vi "ModeloSegundoOrden.vi"() -> ()   [LabVIEW 2019]
uses:
  <vilib>/addons/Control Design/_Model Construction/Special Model Creation.llb/Special Model Creation SubVI/CD Create 2nd Order Model.vi
  <vilib>/addons/Control Design/_Utility/Model Viewer.llb/Model Viewer SubVI/cd_Draw Zero-Pole-Gain Equation (TF).vi
  <vilib>/addons/Control Design/_Utility/Model Viewer.llb/Model Viewer SubVI/cd_Draw Transfer Function Equation (TF).vi
  <vilib>/addons/control/pid/pid.llb/PID (DBL).vi
  <vilib>/addons/control/pid/NI_PID_pid.lvlib
  <vilib>/addons/Control Design/_Model Construction/NI_CD_Special Model Creation.lvlib
  <vilib>/addons/Control Design/_Utility/NI_CD_Model Viewer.lvlib
panel:
  out "Equation 2":picture
  in  "Natural Frequency (rad/s)":dbl format="%.4f"
  in  "stop":bool
  in  "paso (s)":dbl
  in  "PID gains":T1={"proportional gain (Kc)"=1.0, "integral time (Ti, min)"=0.01, "derivative time (Td, min)"=0.0} {"derivative time (Td, min)" format="%.3f"; "integral time (Ti, min)" format="%.3f"; "proportional gain (Kc)" format="%.3f"}
  in  "setpoint":dbl format="%#_13g"
  in  "input cluster":T2
  out "Waveform Chart":T2(graph)
  in  "K":dbl=1.0
  in  "Factor de amortiguamiento":dbl
  out "Equation":picture
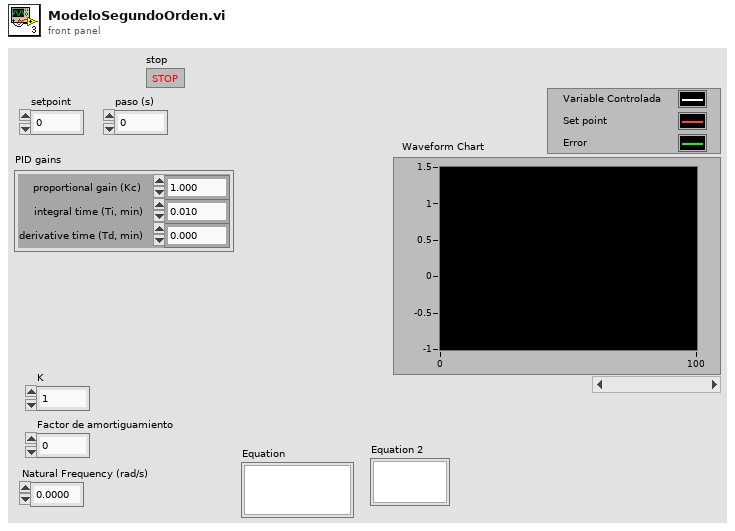
[diagram p1: front panel]
types:
  T1 = cluster{"proportional gain (Kc)":dbl, "integral time (Ti, min)":dbl, "derivative time (Td, min)":dbl}
  T2 = cluster{"Variable controlada":dbl, "Set Point":dbl, "Error":dbl}
  T3 = typedef "NI_LinSys_Model Typedefs.lvlib/CD Transfer Function Model (MIMO).ctl" = cluster{"properties":T4, "transfer function(s)":T5[][]}
  T4 = typedef "NI_LinSys_Model Typedefs.lvlib/CD General Elements.ctl" = cluster{"Model name":string, "Input names":string[], "Output names":string[], "Input Delays":dbl[], "Output Delays":dbl[], "Sampling Time":dbl, "Notes":string}
  T5 = typedef "NI_LinSys_Model Typedefs.lvlib/CD Transfer Function Model (SISO).ctl" = cluster{"Numerator":dbl[], "Denominator":dbl[], "delay":dbl}
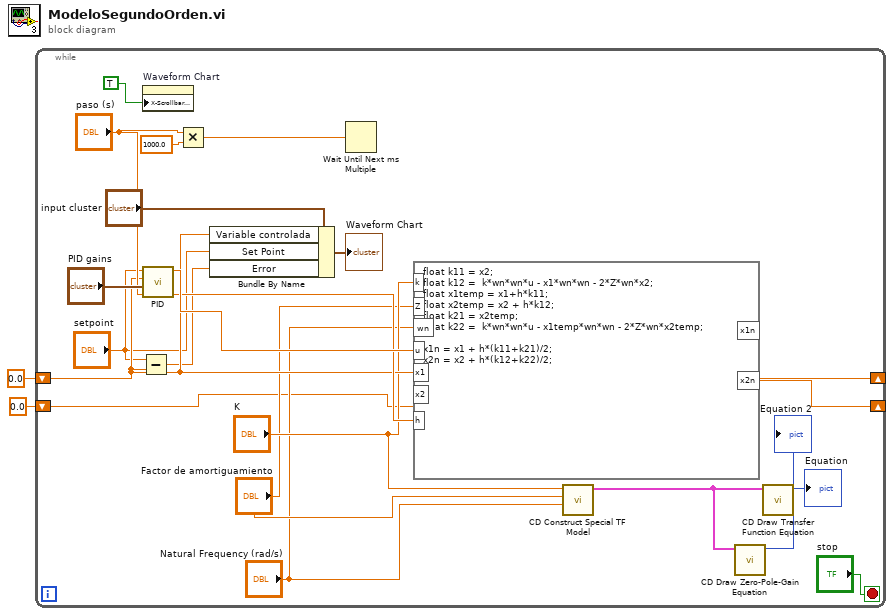
[diagram p0: block diagram]
diagram:
  n1 = while {
    shift-right: [w21] -> _
    shift-left: 0.0 ("xn") -> [w16]
    shift-right: [w6] -> _
    shift-left: 0.0 ("x2n") -> [w5]
    stop <- "stop" stop-if-true
    n2 = Subtract(x="setpoint", y=w16) -> (x-y=w14:dbl)
    n3 = property on="Waveform Chart" class="WFChart (strict)"("X-Scrollbar Visible"=TRUE ("X Scrollbar Visible")) -> ()  [unwired: 2 in, 2 out]
    n4 = call-poly <vilib>:"PID.vi"("dt (s)"="paso (s)", "PID gains"="PID gains", "process variable"=w16, "setpoint"="setpoint") -> ("dt out (s)"=w17:dbl, "output"=w22:dbl)  [unwired: 6 in]
    n5 = Multiply(x="paso (s)", y=1000.0) -> (x*y=w18:dbl)
    n6 = Bundle By Name(cluster="input cluster", "Variable controlada"=w16, "Set Point"="setpoint", "Error"=w14) -> (→"Waveform Chart":T2)
    n7 = Wait Until Next ms Multiple(millisecond multiple=w18) -> ()  [unwired: 1 out]
    n8 = formula code="float k11 = x2;\nfloat k12 =  k*wn*wn*u - x1*wn*wn - 2*Z*wn*x2;\nfloat x1temp = x1+h*k11;\nfloat x2temp = x2 + h*k12;\nfloat k21 = x2temp;\nfloat k22 =  k*wn*wn*u - x1temp*wn*wn - 2*Z*wn*x2temp;\n\nx1n = x1 + h*(k11+k21)/2;\nx2n = x2 + h*(k12+k22)/2;"("k"="K", "Z"="Factor de amortiguamiento", "x1"=w16, "h"=w17, "u"=w22, "wn"="Natural Frequency (rad/s)", "x2"=w5) -> ("x1n"=w21:dbl, "x2n"=w6:dbl)
    n9 = call-poly <vilib>:"CD Construct Special TF Model.vi"("Natural Frequency (rad/s)"="Natural Frequency (rad/s)", "Damping Ratio"="Factor de amortiguamiento", "Static Gain"="K") -> ("Transfer Function Model"=w4:T3)  [unwired: 7 in, 1 out]
    n10 = call-poly <vilib>:"CD Draw Zero-Pole-Gain Equation.vi"("Transfer Function Model"=w4) -> ("Equation"=→"Equation 2":picture)  [unwired: 8 in, 2 out]
    n11 = call-poly <vilib>:"CD Draw Transfer Function Equation.vi"("Transfer Function Model"=w4) -> ("Equation"=→"Equation":picture)  [unwired: 8 in, 2 out]
  }
